vi "Start Or Stop.vi"(7 "timeout":i32=200, 8 "error in (no error)":errorcluster, 9 "AutoStart":bool, 10 "MM Gui Updates In":refnum<queue>, 11 "MM Button Events In":refnum<notifier>) -> (0 "error out":errorcluster, 1 "Start or Stop":T1, 2 "MM Gui Updates Out":refnum<queue>, 3 "Button Events Out":refnum<notifier>)   [LabVIEW 2009]
uses:
  MixedMode/Messages/Mixed Mode Button Events Message.ctl
  MixedMode/Messages/Mixed Mode Button Events.ctl
  Mixed Mode Widget Button States.ctl
  MixedMode/Messages/Mixed Mode Gui Update Msg.ctl
  MixedMode/Messages/Mixed Mode GUI Update Type.ctl
  MixedMode/Messages/Target.ctl
  Data Access Objects/Metadata/LBCB Number.ctl
  Accepted or Declined.ctl
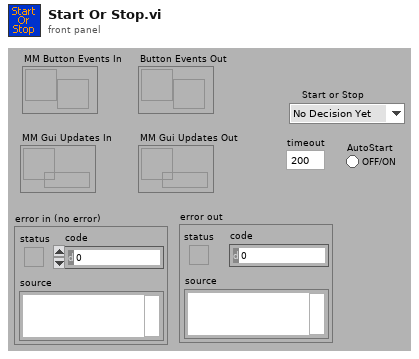
[diagram p1: front panel]
types:
  T1 = typedef "Accepted or Declined.ctl" = enum16{"No Decision Yet", "Accepted", "Declined", "Abort"}
  T2 = typedef "Mixed Mode Gui Update Msg.ctl" = cluster{"MM GUI Update Type":T3, "Targets":T4[], "State":bool, "Step":string}
  T3 = typedef "Mixed Mode GUI Update Type.ctl" = enum16{"Nop", "Targets", "Accept.Blink", "Start.Blink", "TestStats", "Control.Enabled", "StartTestTimer", "RunInputFile", "NTCP Server", "Propose.Auto", "Execute.Auto", "All Autos Off", "Input File Loaded", "Exit"}
  T4 = typedef "Target.ctl" = cluster{"LBCB Number":T5, "DOF Vectors":enum16{" ", "Dx", "Dy", "Dz", "Rx", "Ry", "Rz", "Fx", "Fy", "Fz", "Mx", "My", "Mz"}, "Amount":dbl}
  T5 = typedef "LBCB Number.ctl" = enum16{"LBCB1", "LBCB2"}
  T6 = typedef "Mixed Mode Button Events Message.ctl" = cluster{"MM Control Events":T7, "Button States":T8}
  T7 = typedef "Mixed Mode Button Events.ctl" = enum16{"Propose.Accept", "Propose.Decline", "Execute.Start", "Execute.Stop", "TargetSet", "InputFile.Load", "InputFile.Reset", "InputFile.Pause", "InputFile.Run", "CartesianType.Changed", "NCTP.ConnectToServer", "NTCP.DisconnectFromServer", "Application.Stop", "Control.Enabled", "Control.Disabled", "ControlType.Changed", "Nop"}
  T8 = typedef "Mixed Mode Widget Button States.ctl" = cluster{"Auto-Start Enabled":bool, "Auto-Accept Enabled":bool, "Exit Requested":bool, "Input File Loaded":bool, "Input File Running":bool, "NTCP Server  On":bool}
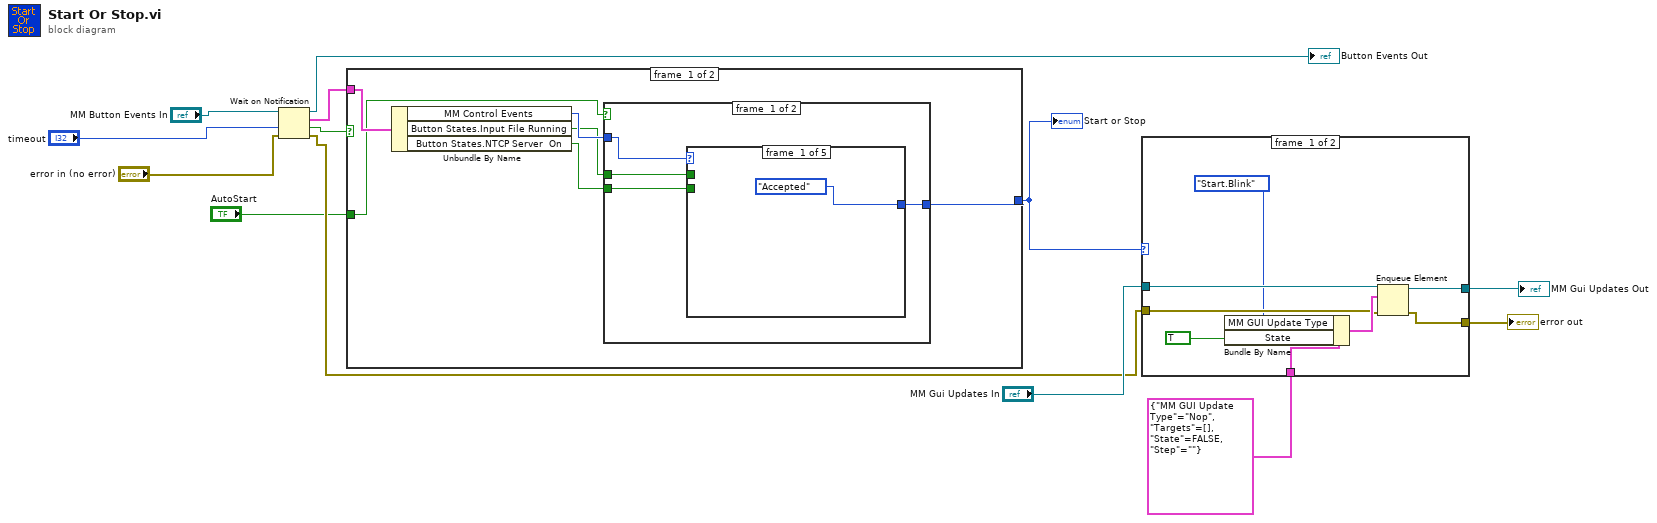
[diagram p0: block diagram]
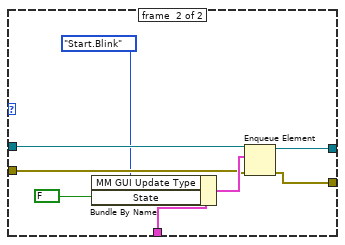
[diagram p2: hidden frame]
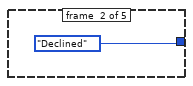
[diagram p3: hidden frame]
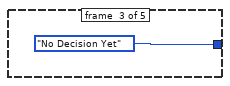
[diagram p4: hidden frame]
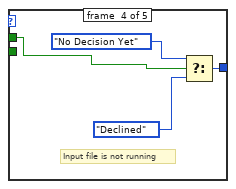
[diagram p5: hidden frame]
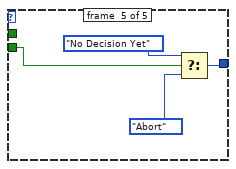
[diagram p6: hidden frame]
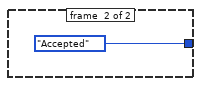
[diagram p7: hidden frame]
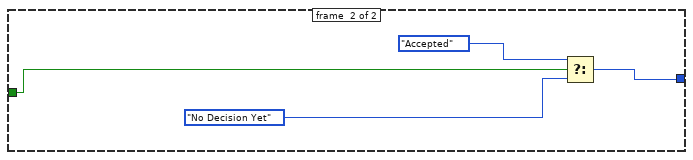
[diagram p8: hidden frame]
diagram:
  n1 = Wait on Notification(notifier="MM Button Events In", timeout in ms (-1)="timeout", error in (no error)="error in (no error)") -> (notifier out=→"Button Events Out":refnum<notifier>, notification=w8:T6, timed out?=w9:bool, error out=w3:errorcluster)  [unwired: 1 in]
  n2 = case shown="False" w9 {
    tunnel: w8 -> [w19 _]
    tunnel: [w17 w38] -> w2
    tunnel: "AutoStart" -> [w16 w37]
    frame #0 {
      n3 = Unbundle By Name(w19) -> ("MM Control Events"=w18:T7, "Button States.Input File Running"=w15:bool, "Button States.NTCP Server  On"=w14:bool)
      n4 = case shown="False" w16 {
        tunnel: w18 -> [w23 _]
        tunnel: [w22 Accepted_or_Declined."Accepted" ("Accepted or Declined")] -> w17
        tunnel: w15 -> [w21 _]
        tunnel: w14 -> [w20 _]
        frame #0 {
          n5 = case shown="\"NTCP.DisconnectFromServer\"" w23 {
            tunnel: [Accepted_or_Declined."Accepted" ("Accepted or Declined") Accepted_or_Declined."Declined" ("Accepted or Declined") Accepted_or_Declined."No Decision Yet" ("Accepted or Declined") w28 w34] -> w22
            tunnel: w21 -> [_ _ _ w27 _]
            tunnel: w20 -> [_ _ _ _ w31]
            frame #0 {
            }
            frame #1 {
            }
            frame #2 {
            }
            frame #3 {
              # "Input file is not running"
              n6 = Select(t=Accepted_or_Declined."No Decision Yet" ("Accepted or Declined"), s=w27, f=Accepted_or_Declined."Declined") -> (s? t:f=w28:T1)
            }
            frame #4 {
              n7 = Select(t=Accepted_or_Declined."No Decision Yet", s=w31, f=Accepted_or_Declined."Abort" ("Accepted or Declined")) -> (s? t:f=w34:T1)
            }
          }
        }
        frame #1 {
        }
      }
    }
    frame #1 {
      n8 = Select(t=Accepted_or_Declined."Accepted", s=w37, f=Accepted_or_Declined."No Decision Yet" ("Accepted or Declined")) -> (s? t:f=w38:T1)
    }
  }
  "Start or Stop" <- w2
  n9 = case shown="\"No Decision Yet\"" w2 {
    tunnel: "MM Gui Updates In" -> [w47 w55]
    tunnel: T2 {"MM GUI Update Type"=enum."Nop", "Targets"=[], "State"=FALSE, "Step"=""} ("element") -> [w46 w54]
    tunnel: [w44 w52] -> w5
    tunnel: [w43 w51] -> w4
    tunnel: w3 -> [w42 w50]
    frame #0 {
      n10 = Bundle By Name(cluster=w46, "MM GUI Update Type"=Mixed_Mode_GUI_Update_Type."Start.Blink", "State"=TRUE) -> (w45:T2)
      n11 = Enqueue Element(queue=w47, element=w45, error in (no error)=w42) -> (queue out=w44:refnum<queue>, error out=w43:errorcluster)  [unwired: 1 in, 1 out]
    }
    frame #1 {
      n12 = Bundle By Name(cluster=w54, "MM GUI Update Type"=Mixed_Mode_GUI_Update_Type."Start.Blink", "State"=FALSE) -> (w53:T2)
      n13 = Enqueue Element(queue=w55, element=w53, error in (no error)=w50) -> (queue out=w52:refnum<queue>, error out=w51:errorcluster)  [unwired: 1 in, 1 out]
    }
  }
  "MM Gui Updates Out" <- w5
  "error out" <- w4
